vi "Accelerate.vi"(8 "error in (no error)":errorcluster, 10 "increment":sgl, 11 "class data in":refnum<class "Ball.lvclass">) -> (0 "error out":errorcluster, 3 "class data out":refnum<class "Ball.lvclass">)   [LabVIEW 2010, in "Labricks.lvlib" / "Ball.lvclass"]
uses:
  Ball.lvclass
  Ball.lvclass/Ball.ctl
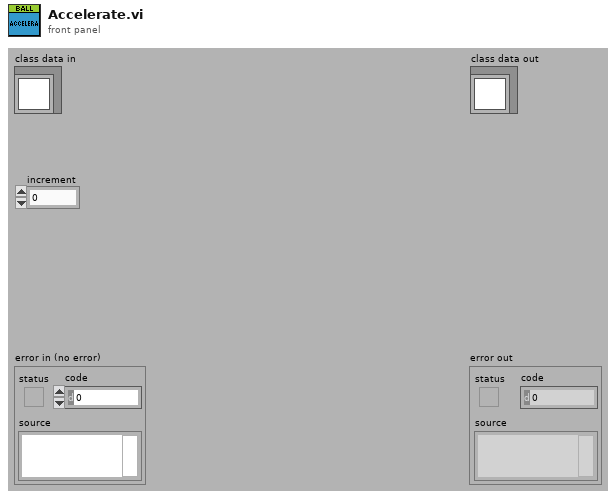
[diagram p1: front panel]
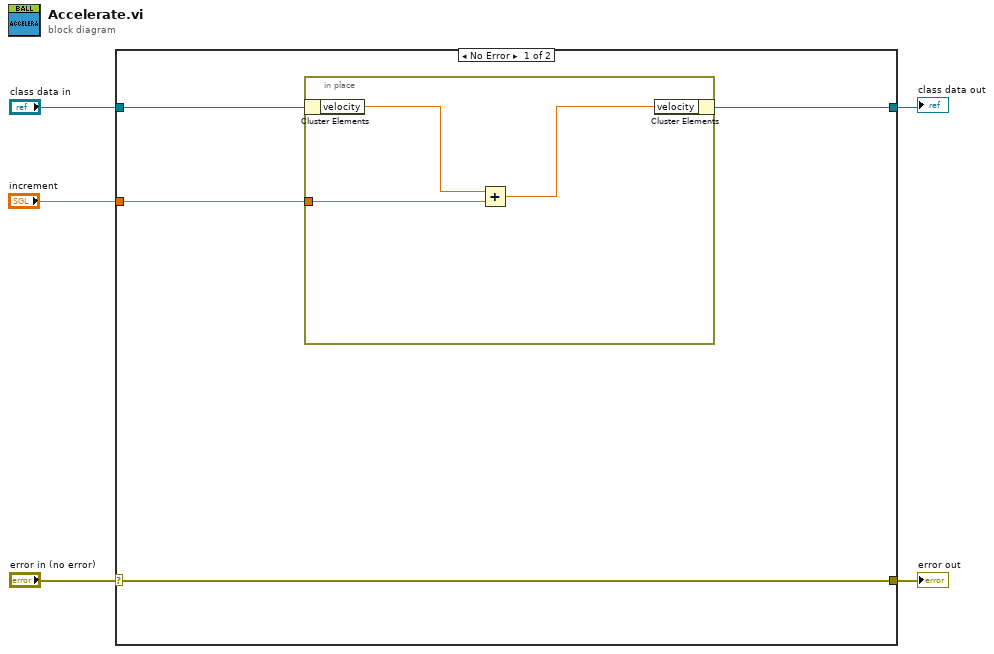
[diagram p0: block diagram]
diagram:
  n1 = case shown="No Error" "error in (no error)" {
    selector: "error in (no error)" -> [w9 w14]
    tunnel: [w9 w14] -> w4
    tunnel: "class data in" -> [w8 w13]
    tunnel: [w7 w13] -> w2
    tunnel: "increment" -> [w6 _]
    frame No Error {
      n2 = in-place {
        in-place-border: w6 -> [w12]
        n3 = in-place-cluster #1(w8) -> ("velocity"=w11:sgl)
        n4 = Add(x=w11, y=w12) -> (x+y=w10:sgl)
        n5 = in-place-cluster #1("velocity"=w10) -> (w7:refnum<class "Ball.lvclass">)
      }
    }
    frame Error {
    }
  }
  "error out" <- w4
  "class data out" <- w2
